vi "LT-FITSDL-HitronicsIQC.vi"(0 "FITSDLL Inputs":T3={"model_type"="Laser Hitronics", "operation"="L000", "revision"="2.10", "dbFITSName"="dbLuminar", "serialnumber"="J24081455", "fsp"=";", "parameters"="SN Hitronics;Machine No.;Result;Remark;Current;Electrical Power;E/O Efficiency;Pump Current;Port 1 Power;Port 2 Power;Port 1 to Port 2 Difference (%);Port 1 Optical Power Setpoint Offset (%);Port 2 Optical Power Setpoint Offset (%);Pulse Width Port 1 (Mean);Pulse Width Port 1 (Min);Pulse Width Port 1 (Max);Pulse Rise Time Port 1 (Mean);Pulse Rise Time Port 1 (Min);Pulse Rise Time Port 1 (Max);Pulse Rise Time Fluctuation Port 1;Pulse Delay Time Port 1 (Mean);Pulse Delay Time Port 1 (Min);Pulse Delay Time Port 1 (Max);Pulse Delay Fluctuation Port 1;Pulse Peak (Mean);Pulse Peak (Min);Pulse Peak (Max);Pulse Peak Fluctuation", "testlabel"="SN Hitronics;Machine No.;Result;Remark;Current;Electrical Power;E/O Efficiency;Pump Current;Port 1 Power;Port 2 Power;Port 1 to Port 2 Difference (%);Port 1 Optical Power Setpoint Offset (%);Port 2 Optical Power Setpoint Offset (%);Pulse Width Port 1 (Mean);Pulse Width Port 1 (Min);Pulse Width Port 1 (Max);Pulse Rise Time Port 1 (Mean);Pulse Rise Time Port 1 (Min);Pulse Rise Time Port 1 (Max);Pulse Rise Time Fluctuation Port 1;Pulse Delay Time Port 1 (Mean);Pulse Delay Time Port 1 (Min);Pulse Delay Time Port 1 (Max);Pulse Delay Fluctuation Port 1;Pulse Peak (Mean);Pulse Peak (Min);Pulse Peak (Max);Pulse Peak Fluctuation", "testresult"="J24081455;DT-FAB-BUILD01;PASS;;310m;19;50;3.19;453.3m;467.7m;-1.72;1.37;3.13;2.063n;1.919n;2.113n;984.5p;762.5p;1.311n;548.8p;92.21n;92.10n;92.40n;300.0p;220.4m;211.1m;230.1m;8.631"}, 7 "FITSDLL Functions":u16(ring) items=["InitDB", "Handshake", "Query", "Log"], 11 "error in (no error)":errorcluster) -> (4 "Response":string, 8 "Response":bool, 15 "FITS  error out":errorcluster)   [LabVIEW 2020]
uses:
  Control 1.ctl
  Control 2.ctl
panel:
  out "Result output":string
  in  "Result":string(combo)="FAIL"
  out "fn_InitDB":string
  in  "FITSDLL._clsDB":refnum<k7>
  # "FITS"
  # "INPUTS"
  # "RESPONSE"
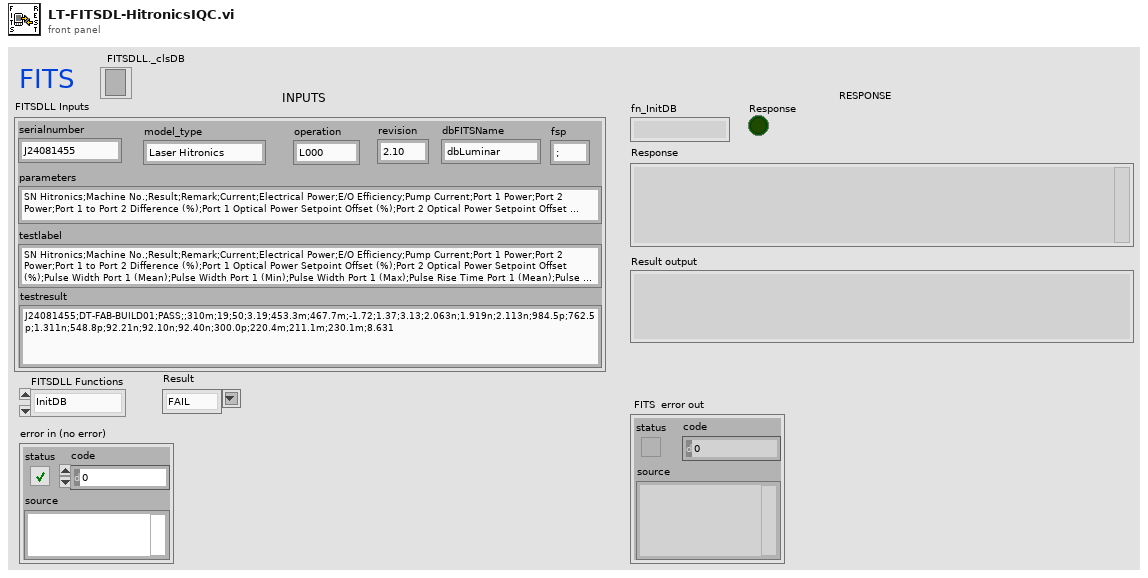
[diagram p1: front panel]
types:
  T1 = typedef "Control 1.ctl" = string
  T2 = typedef "Control 2.ctl" = string
  T3 = cluster{"model_type":string, "operation":string, "revision":string, "dbFITSName":string, "serialnumber":string, "fsp":string, "parameters":T1, "testlabel":string, "testresult":T2}
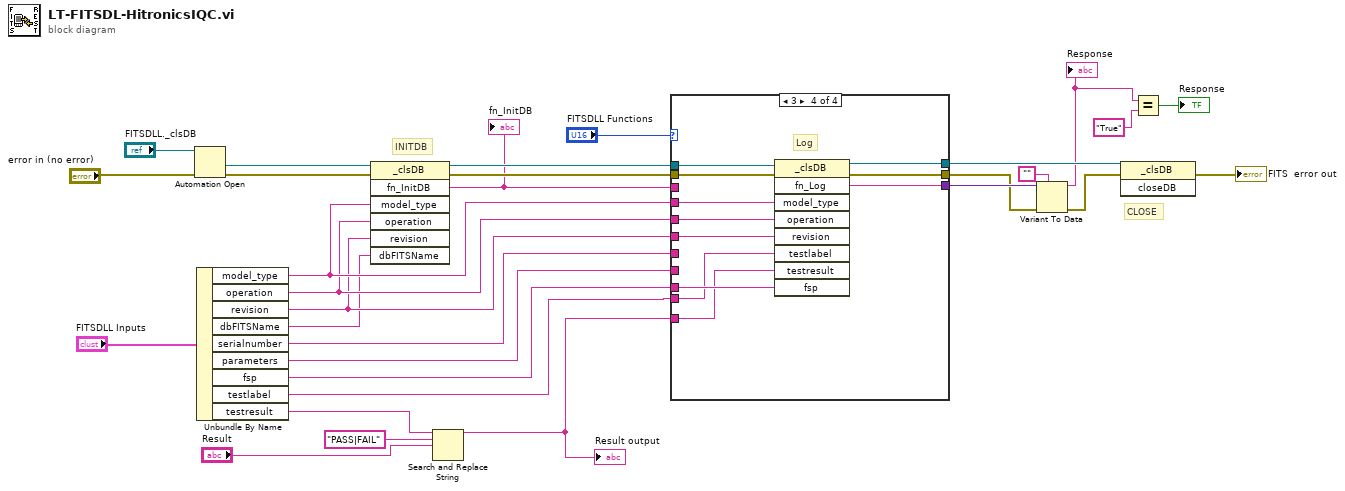
[diagram p0: block diagram]
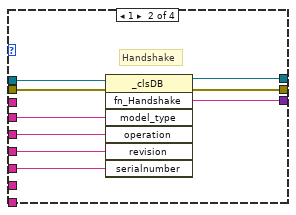
[diagram p3: hidden frame]
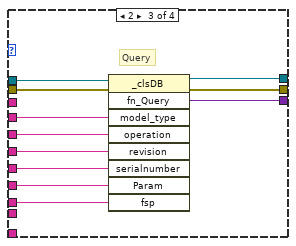
[diagram p4: hidden frame]
diagram:
  # "CLOSE"
  # "INITDB"
  n1 = Automation Open(error in (no error)="error in (no error)", Automation Refnum="FITSDLL._clsDB") -> (Automation Refnum=w27:refnum<k7>, error out=w28:errorcluster)  [unwired: 2 in]
  n2 = Unbundle By Name("FITSDLL Inputs") -> ("model_type"=w22:string, "operation"=w21:string, "revision"=w20:string, "dbFITSName"=w19:string, "serialnumber"=w13:string, "parameters"=w8:T1, "fsp"=w10:string, "testlabel"=w9:string, "testresult"=w5:T2)
  n3 = invoke class="_clsDB" method="fn_InitDB"(reference=w27, error in=w28, "model_type"=w22, "operation"=w21, "revision"=w20, "dbFITSName"=w19) -> (reference out=w26:refnum<k7>, error out=w24:errorcluster, "fn_InitDB"=w11:string)  [unwired: 1 in, 4 out]
  "fn_InitDB" <- w11
  n4 = Search and Replace String(input string=w5, search string="PASS|FAIL", replace string="Result") -> (result string=w4:string)  [unwired: 5 in, 3 out]
  "Result output" <- w4
  n5 = case shown="3" "FITSDLL Functions" {
    tunnel: w26 -> [w33 w42 w53 w55]
    tunnel: [w33 w41 w52 w64] -> w25
    tunnel: w24 -> [w32 w40 w51 w54]
    tunnel: w22 -> [_ w39 w50 w58]
    tunnel: w21 -> [_ w38 w49 w57]
    tunnel: w20 -> [_ w37 w48 w56]
    tunnel: [w31 w36 w47 w63] -> w18
    tunnel: [w32 w35 w46 w62] -> w16
    tunnel: w13 -> [_ w34 w45 _]
    tunnel: w11 -> [w31 _ _ _]
    tunnel: w10 -> [_ _ w44 w61]
    tunnel: w9 -> [_ _ _ w60]
    tunnel: w8 -> [_ _ w43 _]
    tunnel: w4 -> [_ _ _ w59]
    frame 0, Default {
      # "InitDB"
    }
    frame 1 {
      # "Handshake"
      n6 = invoke class="_clsDB" method="fn_Handshake"(reference=w42, error in=w40, "model_type"=w39, "operation"=w38, "revision"=w37, "serialnumber"=w34) -> (reference out=w41:refnum<k7>, error out=w35:errorcluster, "fn_Handshake"=w36:string)  [unwired: 1 in, 4 out]
    }
    frame 2 {
      # "Query"
      n7 = invoke class="_clsDB" method="fn_Query"(reference=w53, error in=w51, "model_type"=w50, "operation"=w49, "revision"=w48, "serialnumber"=w45, "Param"=w43, "fsp"=w44) -> (reference out=w52:refnum<k7>, error out=w46:errorcluster, "fn_Query"=w47:variant)  [unwired: 1 in, 6 out]
    }
    frame 3 {
      # "Log"
      n8 = invoke class="_clsDB" method="fn_Log"(reference=w55, error in=w54, "model_type"=w58, "operation"=w57, "revision"=w56, "testlabel"=w60, "testresult"=w59, "fsp"=w61) -> (reference out=w64:refnum<k7>, error out=w62:errorcluster, "fn_Log"=w63:string)  [unwired: 1 in, 6 out]
    }
  }
  n9 = Variant To Data(error in=w16, type="", Variant=w18) -> (data=w3:string, error out=w15:errorcluster)
  "Response" <- w3
  n10 = invoke class="_clsDB" method="closeDB"(reference=w25, error in=w15) -> (error out=→"FITS  error out":errorcluster)  [unwired: 1 in, 2 out]
  n11 = Equal?(x=w3, y="True") -> (x = y?=→"Response":bool)
